vi "BusTapeAlignment.vi"(6 "Sample Size":dbl=3.0, 8 "um/pix resolution":dbl=1.5800403213058958, 9 "Input Images Array":T2[](array[typedef])=["image_000_-514_122_-18", "image_001_-514_122_-18", "image_002_-514_122_-18", "image_003_-313_122_-18", "image_004_-313_122_-18", "image_005_-313_122_-18", "image_006_-117_122_-18", "image_007_-117_122_-18", "image_008_-117_122_-18", "image_009_79_122_-18", "image_010_79_122_-18", "image_011_79_122_-18", "image_012_275_122_-18", "image_013_275_122_-18", "image_014_275_122_-18", "image_015_471_122_-18", "image_016_471_122_-18", "image_017_471_122_-18", "image_018_667_122_-18", "image_019_667_122_-18", "image_020_667_122_-18"], 10 "Input Coordinate Array":dbl[][](array[numeric])=[[-513.9998637248234, 121.79990691750109, -18.000005000885157], [-513.9997971965031, 121.79999854652941, -18.000005000885157], [-513.9997967387395, 121.80000114052355, -18.000005000885157], [-313.00098288917064, 121.80003348915636, -18.000105000885156], [-312.9997933902692, 121.7999861106163, -18.000005000885157], [-312.99979957007884, 121.79999938576279, -18.000005000885157], [-116.99990596347791, 121.79997588722763, -18.000005000885157], [-116.99979922824845, 121.79999541847765, -18.000005000885157], [-116.99980220371229, 121.7999800071007, -18.000005000885157], [78.99911794644981, 121.79997848122177, -18.000005000885157], [79.00021581632286, 121.7999918326622, -18.000005000885157], [79.00020170194296, 121.79998832314074, -18.000005000885157], [275.0002907429581, 121.79998870461044, -18.000005000885157], [275.00020926102457, 121.79998580544054, -18.000005000885157], [275.00020056351474, 121.79999587624133, -18.000005000885157], [471.0000716463072, 121.7999532279259, -18.000005000885157], [471.0002032533629, 121.79999351112902, -18.000005000885157], [471.0002024141295, 121.79999557106552, -18.000005000885157], [667.001776401648, 121.7999774894005, -18.000005000885157], [667.0002022286744, 121.79999969093859, -18.000005000885157], [667.0002048989625, 121.79999579994738, -18.000005000885157]], 11 "Template Path":path=path "C:/Users/Aerotech/Documents/BNL_ThermomechanicalStave/0_Calibration") -> (0 "Residue":dbl=21890.532329338694, 1 "Bus Tape Positions":cluster{"Top":dbl[], "Top":dbl[]}[](graph)=[{"Top"=[-513.3130412830541, -310.8292165483652, -114.82886039700526, 81.1708205563795, 277.17120892397344, 473.17113450607417, 667.4264678946364], "Top"=[118.76205305390579, 118.76357413135176, 118.76504650437481, 118.76651887232572, 118.76799124559079, 118.76946361537937, 118.77092287962807]}, {"Top"=[-513.3130412830541, -310.8292165483652, -114.82886039700526, 81.1708205563795, 277.17120892397344, 473.17113450607417, 667.4264678946364], "Top"=[120.80859129041323, 118.7663289116045, 118.766306354028, 118.76630879543426, 118.76631271185677, 118.76630335313284, 121.8994406317235]}, {"Top"=[-513.3117559083068, -513.3143266578013, nan, -310.82921586338466, -310.82921723334573, nan, -114.82886033622238, -114.82886045778814, nan, 81.17082118620003, 81.17081992655896, nan, 277.17120897371825, 277.1712088742286, nan, 473.17113458181643, 473.1711344303319, nan, 667.4265226164234, 667.4264131728494, nan, -513.3130412830541, -513.3130412830541, -513.3130412830541, -310.8292165483652, -310.8292165483652, -310.8292165483652, -114.82886039700526, -114.82886039700526, -114.82886039700526, 81.1708205563795, 81.1708205563795, 81.1708205563795, 277.17120892397344, 277.17120892397344, 277.17120892397344, 473.17113450607417, 473.17113450607417, 473.17113450607417, 667.4264678946364, 667.4264678946364, 667.4264678946364], "Top"=[120.80859129041323, 120.80859129041323, 120.80859129041323, 118.7663289116045, 118.7663289116045, 118.7663289116045, 118.766306354028, 118.766306354028, 118.766306354028, 118.76630879543426, 118.76630879543426, 118.76630879543426, 118.76631271185677, 118.76631271185677, 118.76631271185677, 118.76630335313284, 118.76630335313284, 118.76630335313284, 121.8994406317235, 121.8994406317235, 121.8994406317235, 120.81035994636309, 120.80682263446337, nan, 118.7663289360449, 118.76632888716411, nan, 118.76630636432326, 118.76630634373275, nan, 118.76630880235574, 118.76630878851277, nan, 118.76631271704102, 118.76631270667252, nan, 118.76630337700723, 118.76630332925845, nan, 121.89947529408241, 121.89940596936458, nan]}], 2 "Angle (rad)":dbl=7.512093610131177e-06, 3 "Average positions":dbl[][](array[numeric])=[[-513.3130412830541, -310.8292165483652, -114.82886039700526, 81.1708205563795, 277.17120892397344, 473.17113450607417, 667.4264678946364], [120.80859129041323, 118.7663289116045, 118.766306354028, 118.76630879543426, 118.76631271185677, 118.76630335313284, 121.8994406317235]])   [LabVIEW 2016]
uses:
  <vilib>/vision/Image Controls.llb/IMAQ Image.ctl
  <vilib>/vision/Measure.llb/Edge Options.ctl
  <vilib>/vision/Measure.llb/Edge Polarity.ctl
  <vilib>/Analysis/6fits.llb/Curve Fitting Criteria.ctl
  <vilib>/vision/NI_Vision_Development_Module.lvlib
  <vilib>/Analysis/NI_AALPro.lvlib
panel:
  out "pixels y":dbl=1374.0
  out "pixels x":dbl=1920.0
  out "Position errors":dbl[][](array[numeric])=[[1.2853747472697223, 0.0006849805227941929, 6.078288075340342e-05, 0.0006298205356533977, 4.974482246885964e-05, 7.574226556172416e-05, 0.05472178704824274], [1.7686559498535506, 2.44403935651515e-05, 1.0295254739114687e-05, 6.921477099054925e-06, 5.184247037299814e-06, 2.3874397951806625e-05, 0.03466235891451847]]
  in  "Tab Control":T1(tab)=enum."Fit Parameters "
  in  "Coordinate file for image capture":path=path "C:/Users/Aerotech/cernbox/BNL/Stave Assembly Records/2017-04-25/staveCalib/staveCoordinatesSystemCaptured.csv"
  in  "Images Directory":path=path "C:/Users/Aerotech/cernbox/BNL/Stave Assembly Records/2017-04-25/staveCalib"
  in  "Naming Convention":string="image_*_*_*_*.png"
  out "Coordinate array for image capture":dbl[][](array[numeric])=[[-513.9998637248234, 121.79990691750109, -18.000005000885157], [-513.9997971965031, 121.79999854652941, -18.000005000885157], [-513.9997967387395, 121.80000114052355, -18.000005000885157], [-313.00098288917064, 121.80003348915636, -18.000105000885156], [-312.9997933902692, 121.7999861106163, -18.000005000885157], [-312.99979957007884, 121.79999938576279, -18.000005000885157], [-116.99990596347791, 121.79997588722763, -18.000005000885157], [-116.99979922824845, 121.79999541847765, -18.000005000885157], [-116.99980220371229, 121.7999800071007, -18.000005000885157], [78.99911794644981, 121.79997848122177, -18.000005000885157], [79.00021581632286, 121.7999918326622, -18.000005000885157], [79.00020170194296, 121.79998832314074, -18.000005000885157], [275.0002907429581, 121.79998870461044, -18.000005000885157], [275.00020926102457, 121.79998580544054, -18.000005000885157], [275.00020056351474, 121.79999587624133, -18.000005000885157], [471.0000716463072, 121.7999532279259, -18.000005000885157], [471.0002032533629, 121.79999351112902, -18.000005000885157], [471.0002024141295, 121.79999557106552, -18.000005000885157], [667.001776401648, 121.7999774894005, -18.000005000885157], [667.0002022286744, 121.79999969093859, -18.000005000885157], [667.0002048989625, 121.79999579994738, -18.000005000885157]]
  out "Filenames Array":string[](array[string])
  in  "Test?":bool
  in  "Pattern Match Settings":T3={"Algorithm"=2, "Number of Matches Requested"=1, "Minimum Match Score"=700.0, "SubPixel Accuracy"=TRUE, "Rotation Angle Ranges"=[{"Start"=0.0, "End"=360.0}], "Show Search Area"=FALSE, "Show Result"=TRUE} {"Rotation Angle Ranges"."End" format="%.1f"; "Rotation Angle Ranges"."Start" format="%.1f"; "Minimum Match Score" min=0 max=1000 format="%.2f"; "Number of Matches Requested" min=1; "Algorithm" items=["All", "Low Discrepancy Sampling", "Grayscale Value Pyramid", "Gradients Pyramid"]}
  in  "Circle ROI Descriptor":T4={"Global Rectangle"=[675, 567, 1751, 1642], "Contours"=[{"ID"=enum."External", "Type"=7, "Coordinates"=[1212, 1104, 85, 537, 0, 0]}]} {"Contours"."Type" items=["No Selection", "Point", "Line", "Rectangle", "Oval", "Polygon", "Freehand Region", "Annulus", "Unused2", "Unused3", "Broken Line", "Freehand Line", "Rotated Rectangle"]}
  in  "Circle Finding Options":T7={"Search  Direction"=1, "Edge Options"={"Edge Polarity"=2, "Kernel Size"=3, "Width"=3, "Minimum Edge Strength"=10.0, "Interpolation Type"=enum."Bilinear Fixed", "Data Processing Method"=enum."Median"}, "Show Search Area"=FALSE, "Show Search Lines"=FALSE, "Show Edges Found"=FALSE, "Show Result"=TRUE, "Search Area Color"=65280, "Search Lines Color"=255, "Edge Locations Color"=16776960, "Result Color"=65511, "Overlay Group Name"=""} {"Search  Direction" items=["Outside to Inside", "Inside to Outside"]; "Edge Options"."Edge Polarity" items=["All Edges", "Rising Edges", "Falling Edges"]; "Edge Options"."Minimum Edge Strength" format="%.2f"; "Edge Options"."Width" step=2; "Edge Options"."Kernel Size" step=2}
  in  "Circle Fit Options":T8={"Process"=enum."Get Best Edge", "Step Size"=3.0, "Max Pixel Radius"=3}
  in  "Fit Method":T9 items=["Least Square", "Least Absolute Residual", "Bisquare"]
  out "Bus Tape Images":T2[](array[plugin-control])=["image_000_-514_122_-18", "image_001_-514_122_-18", "image_002_-514_122_-18", "image_003_-313_122_-18", "image_004_-313_122_-18", "image_005_-313_122_-18", "image_006_-117_122_-18", "image_007_-117_122_-18", "image_008_-117_122_-18", "image_009_79_122_-18", "image_010_79_122_-18", "image_011_79_122_-18", "image_012_275_122_-18", "image_013_275_122_-18", "image_014_275_122_-18", "image_015_471_122_-18", "image_016_471_122_-18", "image_017_471_122_-18", "image_018_667_122_-18", "image_019_667_122_-18", "image_020_667_122_-18"]
  out "Processing Image #":i32=20
  out "error out":errorcluster
  in  "error in":errorcluster
  out "Template Image":T2
  # "CALIBRATE STAGE ANGLE WITH BUS TAPE  Brandeis University - Brookhaven National Laboratory * ATLAS Phase II Inner Tracker Upgrade"
  # "Overview: This takes a set of images of one row of bus tape circles (seven total) and uses pattern recognition techniques to find the center of the tape at each image. It plots the positions of the centers for each circle and calculates the angle they make in radians. \n \nRequirements: NI Vision Development Module\n\nInstructions: This was created to run in the BuildThermomechanicalStave framework, but it can also be run alone. To do this, input the coordinates of your images, the directory and naming convention of these images, the microns per pixel in these images, the number of each (sample size) and a circle template."
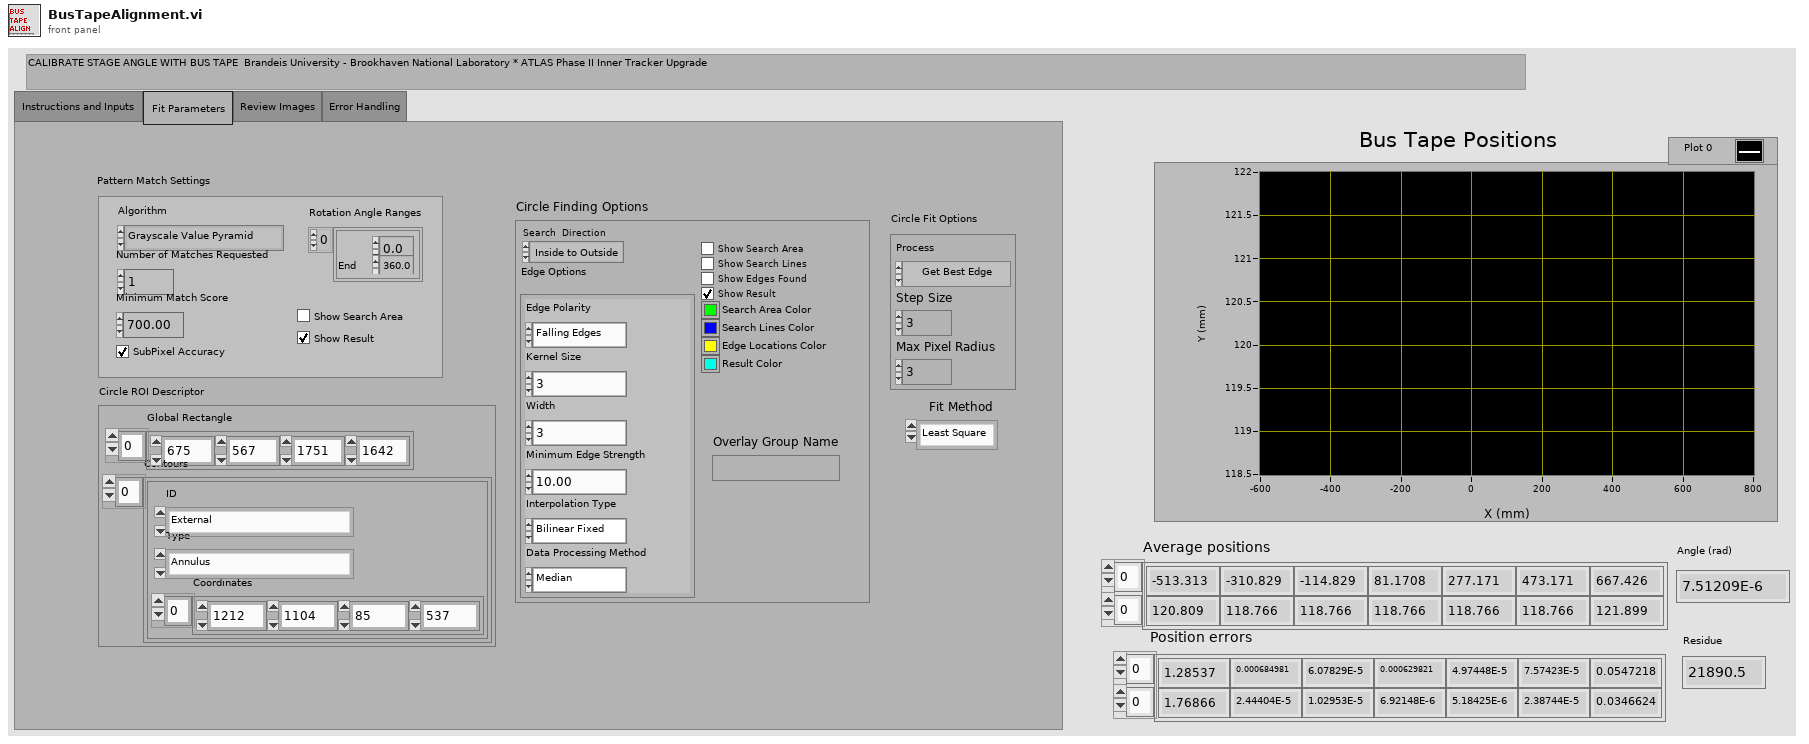
[diagram p1: front panel]
types:
  T1 = enum32{"Instructions and Inputs ", "Fit Parameters ", "Review Images", "Error Handling"}
  T2 = typedef "IMAQ Image.ctl" = refnum<image>
  T3 = cluster{"Algorithm":i32, "Number of Matches Requested":i32, "Minimum Match Score":sgl, "SubPixel Accuracy":bool, "Rotation Angle Ranges":cluster{"Start":sgl, "End":sgl}[], "Show Search Area":bool, "Show Result":bool}
  T4 = cluster{"Global Rectangle":i32[], "Contours":cluster{"ID":enum32{"External", "Internal"}, "Type":u32, "Coordinates":i32[]}[]}
  T5 = typedef "Edge Options.ctl" = cluster{"Edge Polarity":T6, "Kernel Size":u32, "Width":u32, "Minimum Edge Strength":sgl, "Interpolation Type":enum32{"Zero Order", "Bilinear", "Quadratic", "Cubic", "Bilinear Fixed"}, "Data Processing Method":enum32{"Average", "Median"}}
  T6 = typedef "Edge Polarity.ctl" = u32
  T7 = cluster{"Search  Direction":u32, "Edge Options":T5, "Show Search Area":bool, "Show Search Lines":bool, "Show Edges Found":bool, "Show Result":bool, "Search Area Color":u32, "Search Lines Color":u32, "Edge Locations Color":u32, "Result Color":u32, "Overlay Group Name":string}
  T8 = cluster{"Process":enum16{"Get First Edge", "Get First + Last Edge", "Get All Edges", "Get Best Edge"}, "Step Size":dbl, "Max Pixel Radius":i32}
  T9 = typedef "NI_AALPro.lvlib/Curve Fitting Criteria.ctl" = u16
  T10 = cluster{"Position":cluster{"x":sgl, "y":sgl}, "Angle":sgl, "Scale":sgl, "Score":sgl, "Bounding Box":cluster{"x":sgl, "y":sgl}[]}[]
  T11 = cluster{"Global Rectangle":i32[], cluster{"ID":enum32{"External", "Internal"}, "Type":u32, "Coordinates":i32[]}[]}
  T12 = cluster{"Center (Pixels)":cluster{"X":sgl, "Y":sgl}, "Radius (Pixels)":dbl, "Center (Real-World)":cluster{"X":sgl, "Y":sgl}, "Radius (Real-World)":dbl, "Roundness (Real-World)":dbl, "Average Strength":dbl, "Average SNR (dB)":dbl}
  T13 = cluster{"Average positions":dbl[], "Average positions":dbl[]}
  T14 = cluster{"Average positions":dbl[], "Best Linear Fit":dbl[]}
  T15 = cluster{"Average positions":dbl[], "Average positions":dbl[]}[]
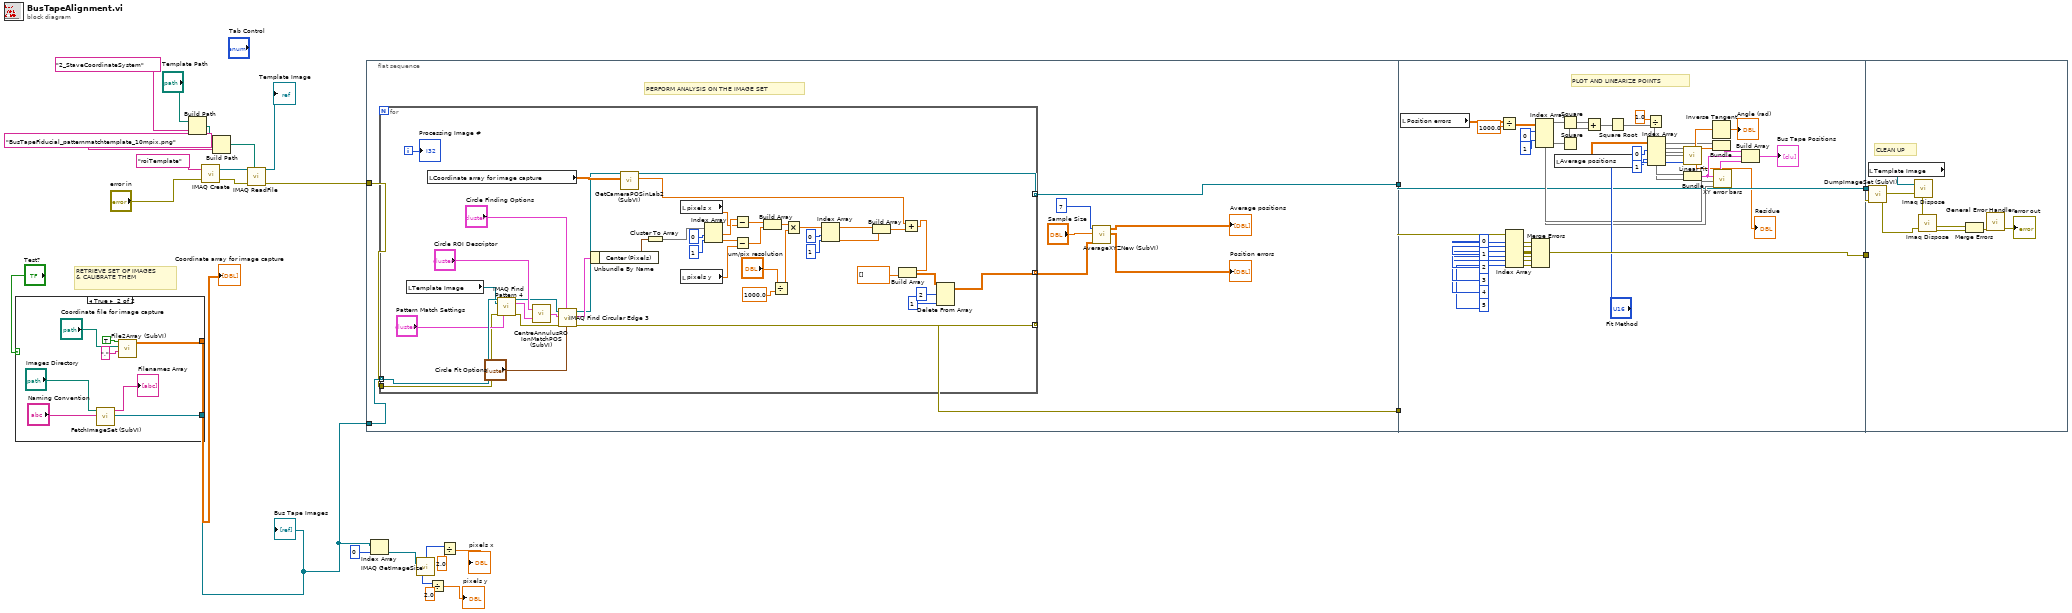
[diagram p0: block diagram]
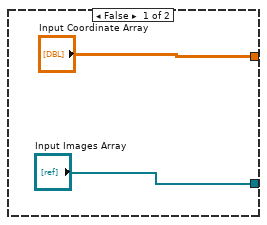
[diagram p2: hidden frame]
diagram:
  # "RETRIEVE SET OF IMAGES\n& CALIBRATE THEM"
  n1 = case shown="True" "Test?" {
    tunnel: ["Input Coordinate Array" w33] -> w21
    tunnel: ["Input Images Array" w29] -> w5
    frame False {
    }
    frame True {
      n2 = call "FetchImageSet (SubVI).vi"("Naming Convention"="Naming Convention", "Images Directory"="Images Directory") -> ("Image Array"=w29:T2[], "Filenames Array"=→"Filenames Array":string[])  [unwired: 7 in, 1 out]
      n3 = call "File2Array (SubVI).vi"("File delimiter"=",", "Source array file"="Coordinate file for image capture", "Load array from file?"=TRUE) -> ("Loaded array"=w33:dbl[][])  [unwired: 7 in, 1 out]
    }
  }
  "Coordinate array for image capture" <- w21
  "Bus Tape Images" <- w5
  n4 = Build Path(base path="Template Path", name or relative path="2_StaveCoordinateSystem") -> (appended path=w15:path)
  n5 = call "IMAQ Create"("Image Name"="roiTemplate", "error in (no error)"="error in") -> ("New Image"=w18:T2, "error out"=w19:errorcluster)  [unwired: 3 in]
  n6 = Build Path(base path=w15, name or relative path="BusTapeFiducial_patternmatchtemplate_10mpix.png") -> (appended path=w13:path)
  n7 = call "IMAQ ReadFile"("File Path"=w13, "error in (no error)"=w19, "Image"=w18) -> ("error out"=w10:errorcluster, "Image Out"=→"Template Image":T2)  [unwired: 4 in, 3 out]
  n8 = flat-sequence {
    tunnel: [w42] -> w25
    tunnel: [w45] -> w24
    tunnel: w5 -> [w44]
    tunnel: w10 -> [w43]
    tunnel: [w95] -> w26
    tunnel: w25 -> [w95]
    tunnel: w24 -> [w130]
    tunnel: [w131] -> w23
    tunnel: w26 -> [w139]
    tunnel: w23 -> [w138]
    frame #0 {
      # "PERFORM ANALYSIS ON THE IMAGE SET"
      n9 = for {
        tunnel: w44 -> [w89] mode=indexing
        tunnel: w43 -> [w87]
        tunnel: [w50] -> w42 mode=indexing
        tunnel: [w80] -> w45 mode=indexing
        tunnel: [w52] -> w38 mode=indexing
        i -> [w74]
        n10 = local read "Template Image"() -> (w79:T2)
        n11 = local read "Coordinate array for image capture"() -> (w69:dbl[][])
        n12 = call "IMAQ Find Pattern 4"("Image"=w89, "Template"=w79, "error in"=w87, "Settings"="Pattern Match Settings") -> ("Image Out"=w77:T2, "Matches (pixel)"=w84:T10, "error out"=w75:errorcluster)  [unwired: 5 in, 4 out]
        n13 = call "CentreAnnulusROIonMatchPOS (SubVI).vi"("Matches (pixel)"=w84, "Annulus ROI Descriptor"="Circle ROI Descriptor") -> ("Annulus ROI Descriptor centred on match position"=w76:T11)
        n14 = call "IMAQ Find Circular Edge 3"("Circle Fit Options"="Circle Fit Options", "Options"="Circle Finding Options", "error in (no error)"=w75, "ROI Descriptor"=w76, "Image"=w77) -> ("error out"=w80:errorcluster, "Fitted Circle"=w68:T12, "Image Out"=w67:T2)  [unwired: 2 in, 2 out]
        n15 = Unbundle By Name(w68) -> ("Center (Pixels)"=w49:cluster{"X":sgl, "Y":sgl})
        n16 = call "GetCameraPOSinLab2 (SubVI).vi"("Loaded array"=w69, "Refnum in"=w67) -> ("Image coordinates in lab frame"=w58:dbl[], "Refnum out"=w50:T2)  [unwired: 7 in, 1 out]
        n17 = Cluster To Array(cluster=w49) -> (array=w63:sgl[])
        n18 = local read "pixels x"() -> (w57:dbl)
        n19 = local read "pixels y"() -> (w59:dbl)
        n20 = Index Array(array=w63, index #1=0 ("index"), index #2=1 ("index")) -> (element #1=w64:sgl, element #2=w60:sgl)
        n21 = Subtract(x=w64, y=w57) -> (x-y=w66:dbl)
        n22 = Subtract(x=w60, y=w59) -> (x-y=w65:dbl)
        n23 = Build Array(w66, w65) -> (w48:dbl[])
        n24 = Divide(x="um/pix resolution", y=1000.0) -> (x/y=w71:dbl)
        n25 = Multiply(x=w48, y=w71) -> (x*y=w83:dbl[])
        n26 = Index Array(array=w83, index #1=0, index #2=1) -> (element #1=w47:dbl, element #2=w46:dbl)
        n27 = Build Array(w47, w46) -> (w70:dbl[])
        n28 = Add(x=w58, y=w70) -> (x+y=w51:dbl[])
        n29 = Build Array(w51, dbl[] [] ("element")) -> (w55:dbl[][])
        n30 = Delete From Array(array=w55, length=2, index (row)=1) -> (array with subset deleted=w52:dbl[][])  [unwired: 1 in, 1 out]
        "Processing Image #" <- w74
      }
      n31 = call "AverageXYZNew (SubVI).vi"("array"=w38, "Number of images each"="Sample Size", "Number of pins"=7) -> ("Uncertainty"=→"Position errors":dbl[][], "Averages"=→"Average positions":dbl[][])  [unwired: 7 in]
    }
    frame #1 {
      # "PLOT AND LINEARIZE POINTS"
      n32 = local read "Position errors"() -> (w112:dbl[][])
      n33 = Divide(x=w112, y=1000.0) -> (x/y=w110:dbl[][])
      n34 = Index Array(array=w130, index #1=0, index #2=1, index #3=2, index #4=3, index #5=4, index #6=5) -> (element #1=w129:errorcluster, element #2=w128:errorcluster, element #3=w127:errorcluster, element #4=w126:errorcluster, element #5=w125:errorcluster, element #6=w124:errorcluster)
      n35 = Merge Errors(w129, w128, w127, w126, w125, w124) -> (w131:errorcluster)
      n36 = Index Array(array=w110, index (row) #1=0, index (row) #2=1) -> (element #1=w109:dbl[], element #2=w103:dbl[])  [unwired: 2 in]
      n37 = local read "Average positions"() -> (w101:dbl[][])
      n38 = Square(x=w109) -> (x^2=w106:dbl[])
      n39 = Square(x=w103) -> (x^2=w104:dbl[])
      n40 = Add(x=w106, y=w104) -> (x+y=w105:dbl[])
      n41 = Square Root(x=w105) -> (sqrt(x)=w107:dbl[])
      n42 = Divide(x=1.0, y=w107) -> (x/y=w108:dbl[])
      n43 = Index Array(array=w101, index (row) #1=0, index (row) #2=1) -> (element #1=w97:dbl[], element #2=w96:dbl[])  [unwired: 2 in]
      n44 = call <vilib>:"Linear Fit.vi"("Y"=w96, "X"=w97, "Weight"=w108, "method"="Fit Method") -> ("Best Linear Fit"=w102:dbl[], "slope"=w99:dbl, "residue"=→"Residue":dbl)  [unwired: 7 in, 2 out]
      n45 = Bundle("Average positions"=w97, "Average positions"=w96) -> (w114:T13)  [unwired: 1 in]
      n46 = Inverse Tangent(1:w99) -> (0:→"Angle (rad)":dbl)
      n47 = Bundle("Average positions"=w97, "Best Linear Fit"=w102) -> (w117:T14)  [unwired: 1 in]
      n48 = call "XY error bars.vi"("XY plot"=w114, "Xerror"=w109, "Yerror"=w103) -> ("X+Y error bars"=w111:cluster{dbl[], dbl[]})  [unwired: 5 in, 2 out]
      n49 = Build Array(w117, w114, w111) -> (→"Bus Tape Positions":T15)
    }
    frame #2 {
      # "CLEAN UP"
      n50 = local read "Template Image"() -> (w137:T2)
      n51 = call "DumpImageSet (SubVI).vi"("error in (no error)"=w138, "Calibrated Image Array"=w139) -> ("error out"=w136:errorcluster)  [unwired: 6 in]
      n52 = call "Imaq Dispose"("Image"=w137, "error in (no error)"=w136) -> ("error out"=w133:errorcluster)  [unwired: 4 in]
      n53 = call "Imaq Dispose"("error in (no error)"=w136) -> ("error out"=w132:errorcluster)  [unwired: 5 in]
      n54 = Merge Errors(w133, w132) -> (w135:errorcluster)
      n55 = call <vilib>:"General Error Handler.vi"("error in (no error)"=w135) -> ("error out"=→"error out":errorcluster)  [unwired: 10 in, 4 out]
    }
  }
  n56 = Index Array(array=w5, index=0) -> (element=w4:T2)
  n57 = call "IMAQ GetImageSize"("Image"=w4) -> ("Y Resolution"=w8:i32, "X Resolution"=w2:i32)  [unwired: 3 in, 1 out]
  n58 = Divide(x=w8, y=2.0) -> (x/y=→"pixels y":dbl)
  n59 = Divide(x=w2, y=2.0) -> (x/y=→"pixels x":dbl)
